vi "Alt Diff Test.vi"() -> ()   [LabVIEW 2013]
panel:
  out "Heading":string
  out "Units":string
  in  "Feet OFF/ Meters ON":bool
  in  "ALT window":bool
  out "O2%":dbl=21.4333 format="%.2f"
  out "Altitude":sgl=1598.218 format="%#.0f"
  in  "West ON/Std OFF":bool
  in  "Set Point Alt":sgl min=0 max=10000 step=1
  out "Alt Dif":dbl(slide)=1598.2180776729308 scale=-1000.0..1000.0 scale format="%.1f"
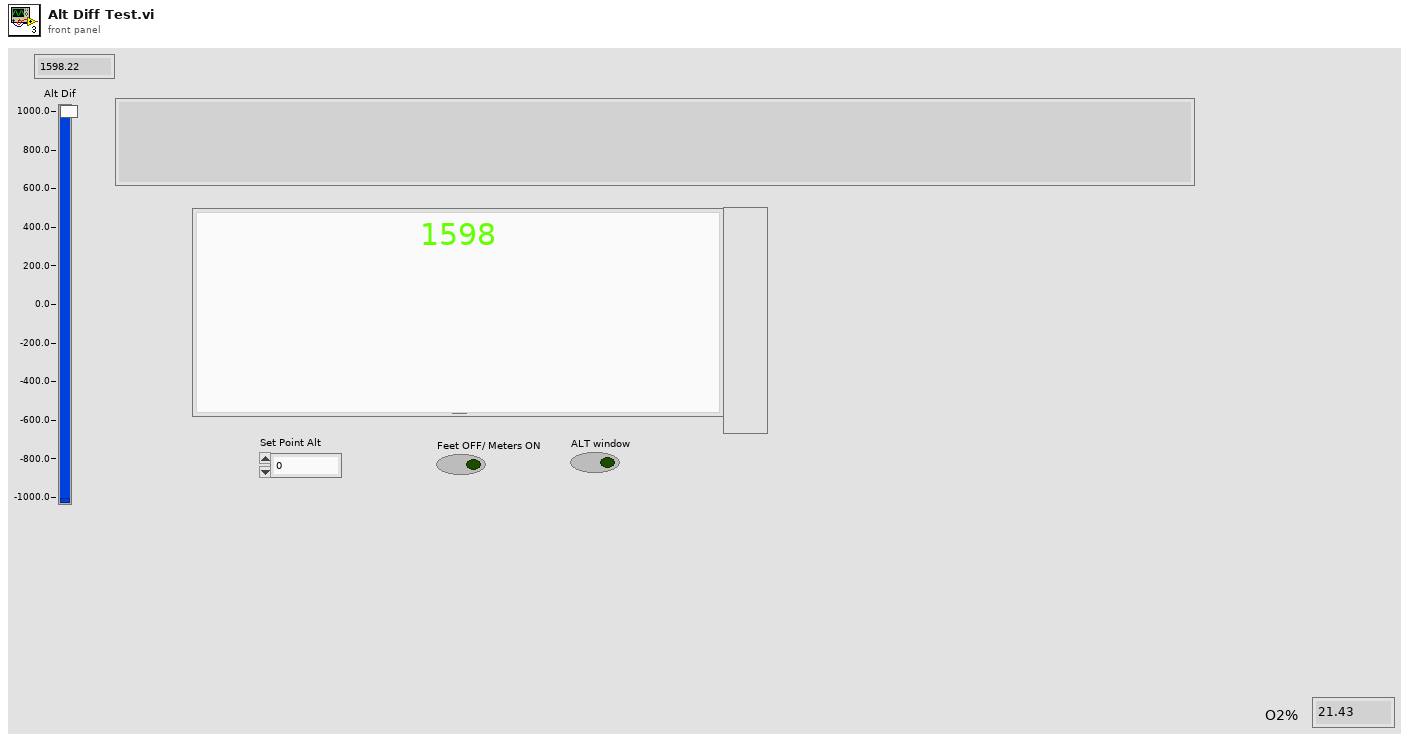
[diagram p1: front panel]
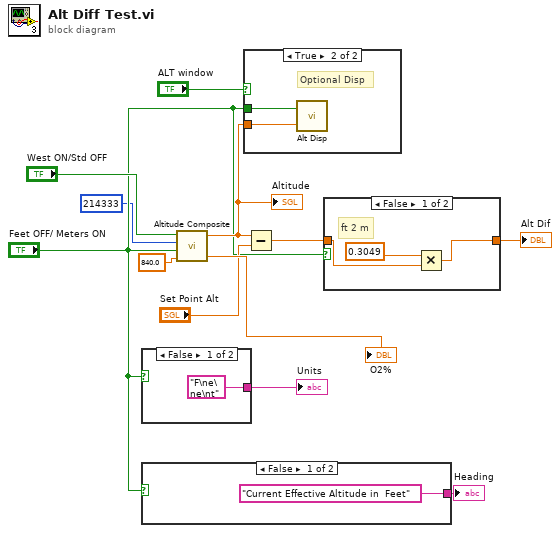
[diagram p0: block diagram]
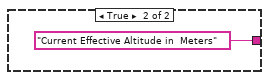
[diagram p2: hidden frame]
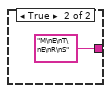
[diagram p4: hidden frame]
diagram:
  n1 = case shown="False" "Feet OFF/ Meters ON" {
    tunnel: ["F\ne\ne\nt" ("Units") "M\nE\nT\nE\nR\nS" ("Units")] -> w8
    frame False {
    }
    frame True {
    }
  }
  "Units" <- w8
  n2 = case shown="False" "Feet OFF/ Meters ON" {
    tunnel: ["Current Effective Altitude in  Feet" ("Heading") "Current Effective Altitude in  Meters" ("Heading")] -> w5
    frame False {
    }
    frame True {
    }
  }
  "Heading" <- w5
  n3 = call "Altitude Composite.vi"("Pressure mBar"=840.0, "Feet OFF/ Meters ON"="Feet OFF/ Meters ON", "O2ppm"=u32 214333, "West ON/Std OFF"="West ON/Std OFF") -> ("O2%"=→"O2%":dbl, "Alt Eff correct"=w9:dbl)  [unwired: 1 out]
  "Altitude" <- w9
  n4 = case shown="True" "ALT window" {
    tunnel: w9 -> [_ w18]
    tunnel: "Feet OFF/ Meters ON" -> [_ w17]
    frame False {
    }
    frame True {
      # "Optional Disp"
      n5 = call "Alt Disp.vi"(2:w18, "Notifer In"=w17) -> ()  [unwired: 2 in]
    }
  }
  n6 = Subtract(x=w9, y="Set Point Alt") -> (x-y=w7:dbl)
  n7 = case shown="False" "Feet OFF/ Meters ON" {
    tunnel: w7 -> [w21 w22]
    tunnel: [w19 w22] -> w6
    frame False {
      # "ft 2 m"
      n8 = Multiply(x=0.3049, y=w21) -> (x*y=w19:dbl)
    }
    frame True {
    }
  }
  "Alt Dif" <- w6
